vi "Write connection reference.vi"(8 "error in (no error)":errorcluster, 10 "reference":T1, 11 "ODBC in":refnum<class "ADODB.lvclass">) -> (0 "error out":errorcluster, 3 "ODBC out":refnum<class "ADODB.lvclass">)   [LabVIEW 2020, in "ADODB.lvclass"]
uses:
  ADODB.lvclass
  <vilib>/addons/database/Connection.llb/Conn ObjectReference.ctl
  ADODB.lvclass/ADODB.ctl
  <vilib>/addons/database/NI_Database_API.lvlib
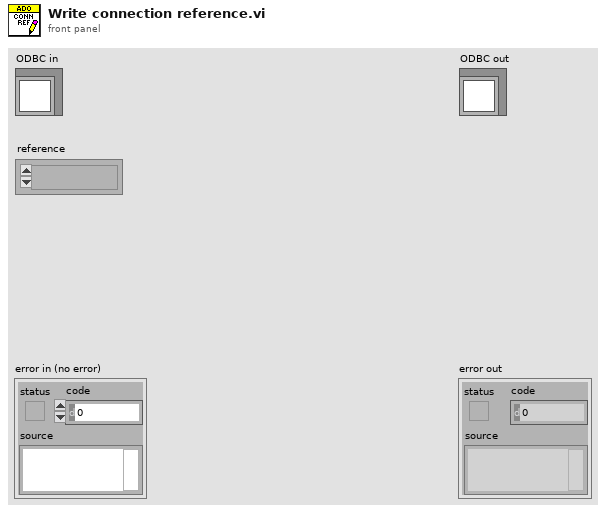
[diagram p1: front panel]
types:
  T1 = typedef "NI_Database_API.lvlib/Conn ObjectReference.ctl" = refnum<k1>
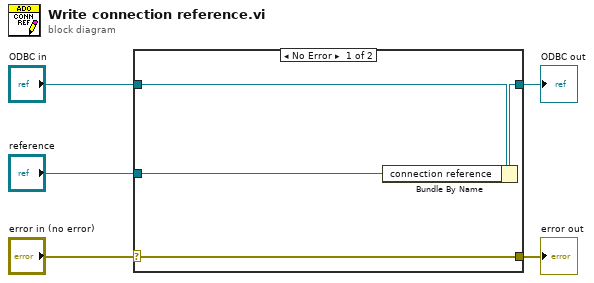
[diagram p0: block diagram]
diagram:
  n1 = case shown="No Error" "error in (no error)" {
    selector: "error in (no error)" -> [w9 w10]
    tunnel: [w9 w10] -> w4
    tunnel: [w7 w11] -> w2
    tunnel: "ODBC in" -> [w8 w11]
    tunnel: "reference" -> [w6 _]
    frame No Error {
      n2 = Bundle By Name(cluster=w8, "connection reference"=w6) -> (w7:refnum<class "ADODB.lvclass">)
    }
    frame Error {
    }
  }
  "error out" <- w4
  "ODBC out" <- w2
